vi "moveAzimuth.vi"(8 "error in (no error)":errorcluster, 10 "azimuth":T1 min=0.0 max=360.0, 11 "DomeController in":refnum<class "DomeController.lvclass">) -> (0 "error out":errorcluster, 3 "DomeController out":refnum<class "DomeController.lvclass">)   [LabVIEW 2016, in "DomeController.lvclass"]
uses:
  DomeController.lvclass
  IDome/domeTypedefs/azimuth.ctl
  domeCommunicator/ComTypedefs/commands.ctl
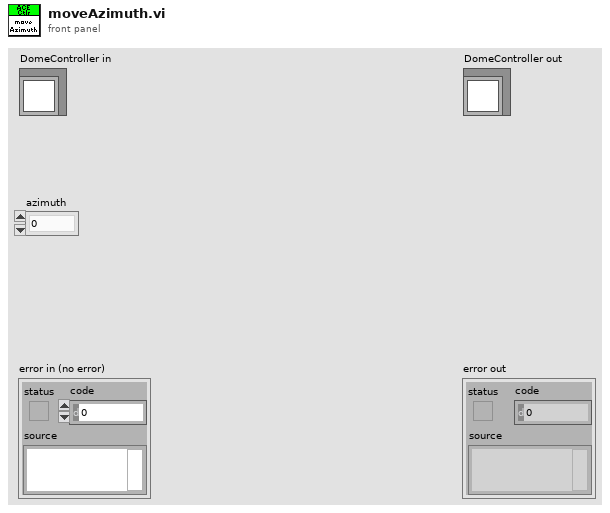
[diagram p1: front panel]
types:
  T1 = typedef "azimuth.ctl" = dbl
  T2 = typedef "commands.ctl" = enum16{"StopAllMotion", "CloseMainDoor", "OpenMainDoor", "CloseDropoutDoor", "OpenDropoutDoor", "SynchronizedOpen", "SynchronizedClose", "AutoShutDownOn", "AutoShutDownOff", "RainOn", "RainOff", "CloudSensorOn", "SloudSensorOff", "RotateToHomePosition", "MoveToAzimuth", "SetTolerance", "DefineHomePosition", "HighSpeedThreshold", "SetCoast", "SetEncoderCountFor360", "SetWatchDogTimer", "SetReverseDirectionMotionDelay", "SaveCurrentConfiguration"}
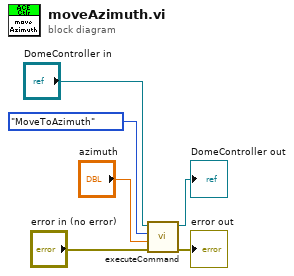
[diagram p0: block diagram]
diagram:
  n1 = call "executeCommand.vi"("error in (no error)"="error in (no error)", "Variant"="azimuth", "commands"=commands."MoveToAzimuth", "DomeController in"="DomeController in") -> ("error out"=→"error out":errorcluster, "DomeController out"=→"DomeController out":refnum<class "DomeController.lvclass">)  [unwired: 6 in]
